vi "Determine Image Path.vi"(11 "image path":path) -> (3 "Path":path)   [LabVIEW 2013, in "DataGrid.lvlib" / "DataGridView.lvclass"]
doc: "Determines the image path for images. If one is passed in and valid, it is used, else the Datagrid folder structure is traversed to find an image path wtih the source files (or executable)."
uses:
  DataGridView.lvclass
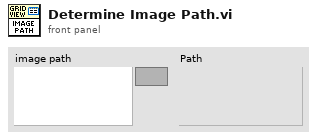
[diagram p1: front panel]
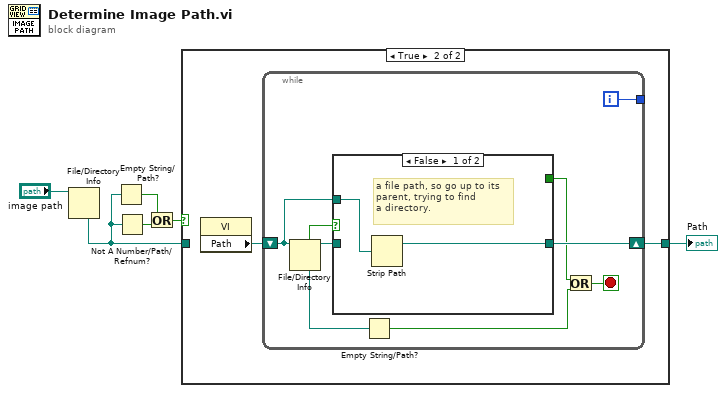
[diagram p0: block diagram]
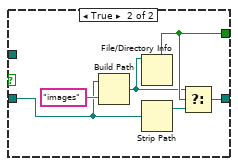
[diagram p3: hidden frame]
diagram:
  n1 = File/Directory Info(path="image path") -> (resolved path=w4:path)  [unwired: 1 in, 6 out]
  n2 = Empty String/Path?(string/path=w4) -> (empty?=w2:bool)
  n3 = Not A Number/Path/Refnum?(number/path/refnum=w4) -> (NaN/Path/Refnum?=w3:bool)
  n4 = Or(x=w2, y=w3) -> (x .or. y?=w1:bool)
  n5 = case shown="True" w1 {
    tunnel: [w7 w8] -> w6
    tunnel: w4 -> [w7 _]
    frame False {
    }
    frame True {
      n6 = property class="VI"() -> ("Path"=w9:path)  [unwired: 2 in, 2 out]
      n7 = while {
        shift-right: [w16] -> w8
        shift-left: w9 -> [w15]
        tunnel: [w12] -> _
        i -> [w12]
        stop <- w13 stop-if-true
        n8 = File/Directory Info(path=w15) -> (path out=w17:path, directory=w18:bool, resolved path=w11:path)  [unwired: 1 in, 4 out]
        n9 = case shown="False" w18 {
          tunnel: w17 -> [_ w22]
          tunnel: [w19 w21] -> w16
          tunnel: [_ w25] -> w14
          tunnel: w15 -> [w20 _]
          frame False {
            # "a file path, so go up to its\nparent, trying to find\na directory."
            n10 = Strip Path(path=w20) -> (stripped path=w19:path)  [unwired: 1 out]
          }
          frame True {
            n11 = Build Path(base path=w22, name or relative path="images") -> (appended path=w24:path)
            n12 = File/Directory Info(path=w24) -> (directory=w25:bool)  [unwired: 1 in, 6 out]
            n13 = Strip Path(path=w22) -> (stripped path=w23:path)  [unwired: 1 out]
            n14 = Select(t=w24, s=w25, f=w23) -> (s? t:f=w21:path)
          }
        }
        n15 = Empty String/Path?(string/path=w11) -> (empty?=w10:bool)
        n16 = Or(x=w14, y=w10) -> (x .or. y?=w13:bool)
      }
    }
  }
  "Path" <- w6
